vi "Init Launch Login.vi"(8 "error in (no error)":errorcluster, 11 "[P] User in":refnum<class "[P] User.lvclass">) -> (0 "error out":errorcluster, 3 "[P] User out":refnum<class "[P] User.lvclass">)   [LabVIEW 2020, in "[P] User.lvlib" / "[P] User.lvclass"]
uses:
  [P] User.lvclass
  [V] Login/[V] Login/[V] Login.lvclass
  <vilib>/ActorFramework/Actor/Actor.lvclass
  C:/Program Files (x86)/National Instruments/LabVIEW 2020/vi.lib/ActorFramework/Actor/Actor.lvclass
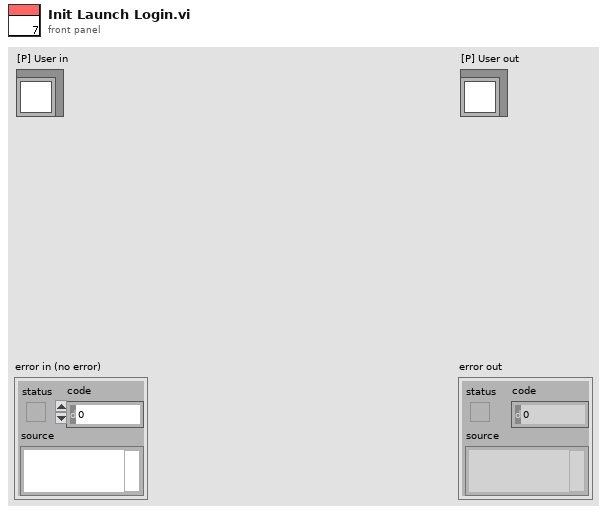
[diagram p1: front panel]
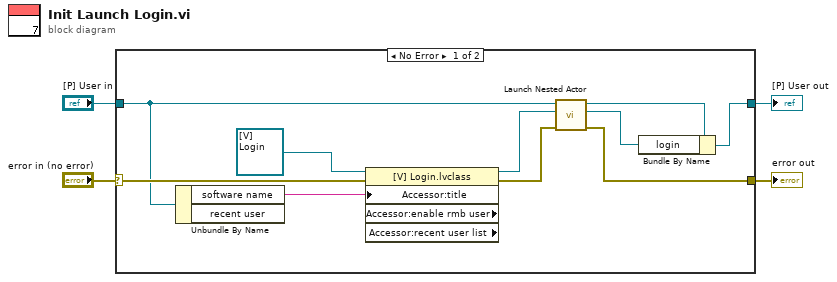
[diagram p0: block diagram]
diagram:
  n1 = case shown="No Error" "error in (no error)" {
    selector: "error in (no error)" -> [w12 w19]
    tunnel: [w7 w19] -> w3
    tunnel: [w8 w18] -> w1
    tunnel: "[P] User in" -> [w11 w18]
    frame No Error {
      n2 = Unbundle By Name(w11) -> ("software name"=w16:string, "recent user"=w17:refnum<class "[Data] Recent User.lvclass">)
      n3 = property class="[V] Login.lvclass"(reference=refnum<class "[V] Login.lvclass"> refnum ("[V] Login.lvlib:[V] Login.lvclass"), error in=w12, "Accessor:title"=w16) -> (reference out=w5:refnum<class "[V] Login.lvclass">, error out=w6:errorcluster, "Accessor:enable rmb user"=w15:bool, "Accessor:recent user list"=w14:string[])
      n4 = call <vilib>:"Launch Nested Actor.vi"("error in (no error)"=w6, "Nested Actor"=w5, "Caller Actor in"=w11) -> ("error out"=w7:errorcluster, "Nested Actor's Enqueuer"=w9:refnum<class "Message Enqueuer.lvclass">, "Caller Actor out"=w10:refnum<class "[P] User.lvclass">)  [unwired: 6 in]
      n5 = Bundle By Name(cluster=w10, "login"=w9) -> (w8:refnum<class "[P] User.lvclass">)
    }
    frame Error {
    }
  }
  "error out" <- w3
  "[P] User out" <- w1
